vi "BonOMM-SAOMM.Test.vi"() -> ()   [LabVIEW 2011] (continued)
  in  "Port Local":u16
  in  "MCB Baud Rate":u32=57600
  out "Warning Code":u32
  in  "ANSW":string
  out "ActiveCmd":T15 caption="Commande Active"
  in  "TCS VRN":refnum<visa-resource-name>="COM7" caption="ID de connexion WinTCS"
  in  "PrAMS VRN":refnum<visa-resource-name>="COM4" caption="ID de connexion PrAMS"
  in  "MC-BonOMM VRN":refnum<visa-resource-name>="COM3"
  out "MCB COMM":bool=TRUE
  out "TCS COMM":bool=TRUE
  out "CmdPending":bool caption="Commande Active ?"
  out "CmdFIFO":T14(array[cluster]) caption="Commandes Latentes"
  out "Error Code":u32
  out "path_exclusion":path=path "C:/BonOMM/BonOMM 7.1/systemlogfiles" caption="Chemin du fichier d'exclusion"
  out "VI principal":path=path "C:/BonOMM/BonOMM 7.1/BonOMM 7.1.vi" caption="Chemin du dossier principal"
  out "path_config":path=path "C:/BonOMM/BonOMM 7.1/BonOMM 7.1.vi" caption="Répertoire de configuration"
  out "properties.ini":path=path "C:/BonOMM/BonOMM 7.1/BonOMM 7.1.vi" caption="Fichier de Configuration Système"
  out "instruments.ini":path=path "C:/BonOMM/BonOMM 7.1/BonOMM 7.1.vi" caption="Paramètres Instrumentaux"
  out "path_data":path=path "C:/BonOMM/BonOMM 7.1/systemlogfiles" caption="Répertoire de données"
  out "path_dss":path=path "C:/BonOMM/BonOMM 7.1/systemlogfiles" caption="Répertoire des données DSS"
  out "path_libdir":path=path "C:/BonOMM/BonOMM 7.1/systemlogfiles" caption="Répertoire des librairies d'objets"
  out "loaded_lib":path=path "C:/BonOMM/BonOMM 7.1/systemlogfiles" caption="Chemin vers la librairie chargée"
  out "path_SubVIs":path=path "C:/BonOMM/BonOMM 7.1/systemlogfiles" caption="Répertoire principal des sous routines"
  out "path_syslogs":path=path "C:/BonOMM/BonOMM 7.1/systemlogfiles" caption="Répertoire d'archivages principal"
  out "path_focuslog":path=path "C:/BonOMM/BonOMM 7.1/systemlogfiles" caption="Répertoire d'archivages des foyers instrumentaux"
  out "path_pointing":path=path "C:/BonOMM/BonOMM 7.1/systemlogfiles" caption="Répertoire d'archivages des pointés"
  out "path_trackfile":path=path "C:/BonOMM/BonOMM 7.1/tracklogfiles" caption="Répertoire d'archivage du guidage"
  out "path_Apps":path=path "C:/BonOMM/BonOMM 7.1/systemlogfiles" caption="Répertoire principal des applications externes"
  out "wgetexec":path=path "C:/BonOMM/BonOMM 7.1/systemlogfiles" caption="Chemin vers l'application wget.exe"
  out "IDLexec":path=path "C:/BonOMM/BonOMM 7.1/systemlogfiles" caption="Chemin vers l'application IDL"
  out "PrAMS COMM":bool=TRUE
  in  "Address du serveur":string
  out "Clients":string[](array[string]) caption="Clients TCP/IP"
  out "Clients ID":refnum<k5>[](array[refnum])
  in  "Hexapod VRN":refnum<visa-resource-name>="COM4" caption="ID de la connexion Hexapod Console"
  out "Calib COMM":bool=TRUE
  out "Calib VRN":refnum<visa-resource-name>="COM5" caption="Visa Ressource Name des lampes"
  in  "Calib Baud rate":u32=9600
  out "ExCmd COMM":bool=TRUE
  in  "Excmd VRN":refnum<visa-resource-name>="COM8"
  in  "Excmd Baud rate":u32=38400
  in  "Table Baud rate":u32=38400 caption="Baud Rate des tables"
  out "Table VRN":refnum<visa-resource-name>="COM9" caption="Visa Ressource Name des tables"
  out "TableCOM":bool=TRUE caption="Tables COMM"
  # "Paramètres"
  # "Control Emulation"
  # "Debug"
  # "Région d'intérêt"
  # "Tables de guidage"
  # "Foyers Télescope/Tables"
  # "Communications"
  # "Guidage"
  # "Falcon Processed"
  # "Position Hexapode"
  # "Position Nominale"
  # "Historique"
  # "X"
  # "Y"
  # "Z"
  # "U"
  # "V"
  # "Commandes"
  # "Offsets"
  # "Gains"
  # "Enabling Tab"
  # "Flags d'états"
  # "Variable d'applications"
  # "Propriétés de la fenêtre"
  # "Logs & Archives"
  # "Utilité à confirmer ..."
  # "Gestion des menus et librairies"
  # "Sauvegarde des Ctrls&Indics"
  # "Lampes de Calibration"
  # "Roues à Filtres"
  # "Caméra d'acquisition"
  # "Station Météo"
  # "Athermalisation des Foyers"
  # "LVDTs"
  # "À passer en commande de menu ..."
  # "Centre du Champ"
  # "TCS Status Bytes"
  # "Data USNO"
  # "À passer en commandes\ndu menu ..."
  # "Télescope (TCS & StarryNight)"
  # "Image de fond"
  # "Coordonnées Relatives"
  # "Centre du champ"
  # "Données USNO"
  # "Image DSS"
  # "Best Target"
  # "Bundles d'erreur"
  # "Temps d'exécution"
  # "Foyer"
  # "Prêt à pointer"
  # "En déplacement"
  # "Temps Univ."
  # "Entrainement"
  # "Temps Sidé."
  # "Angle Hor."
  # "Asc. Droite"
  # "Déclinaison"
  # "Époque"
  # "Air Mass"
  # "Télescope"
  # "Cible"
  # "Référence"
  # "OFFSET"
  # "Curseur"
  # "Z"
  # "Foyer (z)"
  # "X"
  # "Y"
  # "Z"
  # "U"
  # "V"
  # "Position"
  # "Écart"
  # "RA"
  # "DEC"
  # "Total"
  # "Sonde"
  # "Cible"
  # "Exposition"
  # "X"
  # "Y"
  # "Centroïds"
  # "Pixels"
  # "Résidu"
  # "''"
  # "Tmp(°)"
  # "Hum(%)"
  # "Ext."
  # "Int."
  # "Mir."
  # "Str."
  # "RA"
  # "DEC"
  # "Communications"
  # "Commandes Externes"
  # "Chemins système"
  # "Clients TCP/IP"
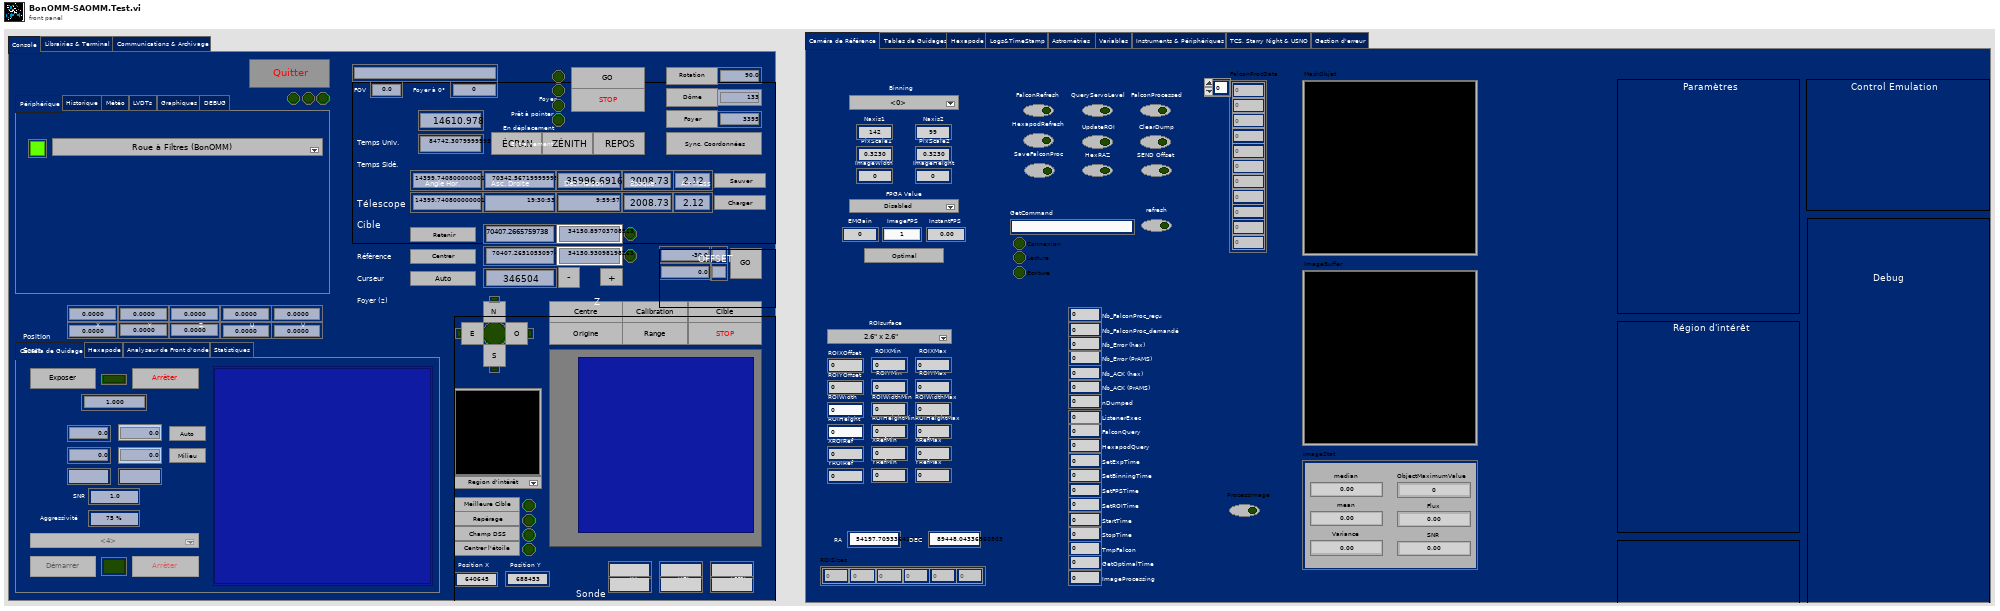
[diagram p1: front panel]
types:
  T1 = enum32{"Caméra de Référence", "Tables de Guidages", "Hexapode", "Logs&TimeStamp", "Astrométries", "Variables", "Instruments & Périphériques", "TCS, Starry Night & USNO", "Gestion d'erreur"}
  T2 = cluster{"median":dbl, "mean":dbl, "Variance":dbl, "ObjectMaximumValue":dbl, "Flux":dbl, "SNR":dbl}
  T3 = cluster{"Command Error":bool, "Slip/Stall":bool, "Overtravel":bool, "Done":bool, "nError":u32, "nSlip":u32, "nOT":u32, "nDone":u32}
  T4 = cluster{"NAXIS":dbl[], "CD":dbl[][], "CDELT":dbl[], "CRPIX":dbl[], "CTYPE":string[], "CRVAL":dbl[], "LONGPOLE":dbl, "LATPOLE":dbl, "PV2":dbl[]}
  T5 = typedef "LVPointTypeDef.ctl" = cluster{"Horizontal":i16, "Vertical":i16}
  T6 = typedef "LVRectTypeDef.ctl" = cluster{"Left":i16, "Top":i16, "Right":i16, "Bottom":i16}
  T7 = cluster{"Source":string, "Error Code":u32, "Warning Code":u32, "Comment":string}[]
  T8 = enum32{"Console", "Librairies & Terminal", "Communications & Archivage"}
  T9 = enum32{"Caméra de Guidage", "Hexapode", "Analyseur de Front d'onde", "Statistiques"}
  T10 = cluster{"X Values":dbl[], "Histogram: h(x)":i32[]}[]
  T11 = enum32{"Périphérique", "Historique", "Météo", "LVDTs", "Graphiques", "DEBUG"}
  T12 = cluster{"filtre #1":bool, "filtre #2":bool, "filtre #3":bool, "filtre #4":bool, "filtre #5":bool, "filtre #6":bool}
  T13 = cluster{"[Temp 1]":dbl, "[Temp 2]":dbl, "[Temp 3]":dbl, "[Temp 4]":dbl, "[Temp 5]":dbl, "[Temp 6]":dbl, "[Temp 7]":dbl, "[Temp 8]":dbl}
  T14 = cluster{"CmdAct":string, "CmdArgs":string, "Source":string}[]
  T15 = cluster{"CmdAct":string, "CmdArgs":string, "Source":string}
  T16 = enum32{"Console", "Librairies & Terminal", "Communications & Archivage", "Secondaire Actif"}
  T17 = enum8{"Enabled", "Disabled", "Disabled and Grayed Out"}
  T18 = cluster{"Source":string, "Error Code":i32, "Warning Code":i32, "Comment":string}[]
  T19 = cluster{"Command Error":bool, "Slip/Stall":bool, "Overtravel":bool, "Done":bool, "nError":dbl, "nSlip":dbl, "nOT":dbl, "nDone":dbl}
  T20 = cluster{"Invert Angle":bool, "Invert X":bool, "Invert Y":bool}
  T21 = cluster{"North Task":refnum<k21>, "West Task":refnum<k21>, "South Task":refnum<k21>, "East Task":refnum<k21>}
  T22 = cluster{"newFoyer":dbl, "updSonde":bool, "oldFoyer":dbl}
  T23 = cluster{"cRIO address":string, "Port Number":u16, "cRIO_commID":refnum<k5>, "Cx":bool}
  T24 = typedef "NI_LVConfig.lvlib/Config Data RefNum.ctl" = refnum<k1>
  T25 = cluster{"left":i16, "top":i16, "right":i16, "bottom":i16}
  T26 = typedef "LVRangeTypeDef.ctl" = cluster{"Minimum":dbl, "Maximum":dbl, "Increment":dbl, "Minor Increment":dbl, "Start":dbl}
  T27 = cluster{"PrAMS VRN":refnum<visa-resource-name>, "Signature":u32, "MessageType":cluster{string[], u32[]}, "Hexapod VRN":refnum<visa-resource-name>}
  T28 = cluster{"HexX":refnum<vi>, "HexY":refnum<vi>, "HexZ":refnum<vi>, "HexU":refnum<vi>, "HexV":refnum<vi>}
  T29 = cluster{"Angle Hor.":refnum<vi>, "DEC Tel":refnum<vi>, "Epoch Tel":refnum<vi>}
  T30 = cluster{"PrAMS actif":refnum<vi>, "PrAMS-ACK":refnum<vi>, "HexaCons actif":refnum<vi>, "Hexapod-ACK":refnum<vi>}
  T31 = cluster{"Offset X":refnum<vi>, "Offset Y":refnum<vi>, "Offset Z":refnum<vi>, "Offset U":refnum<vi>, "Offset V":refnum<vi>}
  T32 = cluster{"Calibration X":dbl, "Calibration Y":dbl}
  T33 = cluster{"Rangement X":dbl, "Rangement Y":dbl, "Rangement Z":dbl}
  T34 = cluster{"Calibration Y":dbl, "Calibration X":dbl}
  T35 = cluster{"Range Y":dbl, "Range X":dbl, "Range Z":dbl}
  T36 = cluster{"Cible X":refnum<vi>, "Cible Y":refnum<vi>, "Cible Z":refnum<vi>}
  T37 = cluster{"Table VRN":refnum<vi>, "Table Error":refnum<vi>, "Table actif":refnum<vi>}
  T38 = typedef "LVMouseTypeDef.ctl" = cluster{"Mouse Position":cluster{"X":i32, "Y":i32}, "Mouse Modifiers":cluster{"Button Down":bool, "Shift Mod":bool, "Menu Mod":bool, "Option Mod":bool}}
  T39 = typedef "LVBoundsTypeDef.ctl" = cluster{"Width":u32, "Height":u32}
  T40 = cluster{"TableAstrom":cluster{"NAXIS":dbl[], "CD":dbl[][], "CDELT":dbl[], "CRPIX":dbl[], "CTYPE":string[], "CRVAL":dbl[], "LONGPOLE":dbl, "LATPOLE":dbl, "PV2":dbl[]}, "FieldAstrom":cluster{"NAXIS":dbl[], "CD":dbl[][], "CDELT":dbl[], "CRPIX":dbl[], "CTYPE":string[], "CRVAL":dbl[], "LONGPOLE":dbl, "LATPOLE":dbl, "PV2":dbl[]}, "GuiderAstrom":cluster{"NAXIS":dbl[], "CD":dbl[][], "CDELT":dbl[], "CRPIX":dbl[], "CTYPE":string[], "CRVAL":dbl[], "LONGPOLE":dbl, "LATPOLE":dbl, "PV2":dbl[]}}
  T41 = cluster{"TCS VRN":refnum<visa-resource-name>, "TCS Error":errorcluster, "Table VRN":refnum<visa-resource-name>, "Table Error":errorcluster}
  T42 = cluster{"TCS actif":refnum<vi>, "Table actif":refnum<vi>, "Position Z":refnum<vi>, "StartServo":refnum<vi>, "Mode":refnum<vi>, "Servo":refnum<vi>, "StopServo":refnum<vi>, "DiffX":refnum<vi>, "DiffY":refnum<vi>, "SNR":refnum<vi>, "MovingXY":refnum<vi>}
  T43 = typedef "LVRowAndColumnTypeDef.ctl" = cluster{"Row":i32, "Column":i32}
  T44 = typedef "LVPointDoubleTypeDef.ctl" = cluster{"Cursor X":dbl, "Cursor Y":dbl}
  T45 = cluster{"name":string, "type desc":i16[], "flat data":string}[]
  T46 = typedef "gfitsio.lvlib/gfitsio-refnum.ctl" = refnum<k1>
  T47 = cluster{"Miroir":dbl, "Cursor.Cursor X":dbl, "Cursor.Cursor Y":dbl, "MirVig":dbl}
  T48 = typedef "LVPoint32TypeDef.ctl" = cluster{"Horizontal":i32, "Vertical":i32}
  T49 = cluster{"ROIXOffset OUT":u16, "ROIYOffset OUT":u16, "ROIWidth OUT":u16, "ROIHeight OUT":u16}
  T50 = cluster{"ROIXMin":u16, "ROIYXMax":u16, "ROIYMin":u16, "ROIYMax":u16}
  T51 = cluster{"ROIXOffset":u16, "ROIYOffset":u16, "ROIWidth":u16, "ROIHeight":u16}
  T52 = cluster{"Largeur de l'image":dbl, "Hauteur de l'image":dbl, "Bits par Pixel":dbl, "ID de l'image":u32, "Frame Rate":dbl, "Largeur de Bande":dbl, "Time Stamp":u64}
  T53 = cluster{"Largeur de la ROI":u16, "Hauteur de la ROI":u16, "Position X de la ROI":u16, "Position Y de la ROI":u16, "Minimum de la ROI":u32, "Maximum de la ROI":u32}
  T54 = cluster{"Seuil du masque":dbl, "Flux":dbl, "SNR":dbl, "Centroide X":dbl, "Centroide Y":dbl}
  T55 = cluster{"Logging ID":u32, "Logging TimeStapmp":u64, "Azimuth":dbl, "Elevation":dbl, "Rotation":dbl, "ServoLevel":u16, "ROIWidth":u16, "ROIHeight":u16, "ROIXOffset":u16, "ROIYOffset":u16, "Pixel X":dbl, "Pixel Y":dbl, "ImageTimeStamp":u64, "CommandTimeStamp":u64, "Flux":dbl, "SNR":dbl, "SNRTreshold":dbl, "CentroidX":dbl, "CentroidY":dbl}
  T56 = cluster{"Hexapod_Nominal":dbl[], "Hexapod_Offset":dbl[], "Hexapod_LUT":dbl[], "Hexapod_ServoX":dbl[], "Hexapode_ServoY":dbl[], "Hexapod_Console":dbl[], "Hexapod_Position":dbl[], "Hexapod_Command":dbl[], "Hexapod_Filtered":dbl[]}
  T57 = cluster{"SNR":dbl, "SNRTreshold":dbl, "Flux":dbl}
  T58 = cluster{"ServoLevel":u16, "ROIXOffset":u16, "CentroidX":dbl, "Pixel X":dbl, "ROIYOffset":u16, "CentroidY":dbl, "Pixel Y":dbl}
  T59 = enum16{"Left Button", "Center Button", "Right Button", "Window Close"}
  T60 = cluster{"GuidingCancel":refnum<vi>, "GuideNorth":refnum<vi>, "GuideSouth":refnum<vi>, "GuideEast":refnum<vi>, "GuideWest":refnum<vi>}
  T61 = cluster{"Commande":string, "Chaîne d'arguments":string, "Source":string}[]
  T62 = cluster{"Source":string, "Error Code":u32, "Warning Code":u32, "Comment":string}
  T63 = enum16{"fractional", "engineering", "exponential"}
  T64 = typedef "event.ctl" = cluster{"message":string, "data":variant}
diagram:
  # "Boucle principale: 8"
  # "Go on?"
  n1 = stacked-sequence {
    seq-local: [_ _ w80 _ _ _ _ _ _ _] -> [_ _ _ w203 w576 w714 w767 w800 w943 w7396]
    seq-local: [_ _ _ w201 _ _ _ _ _ _] -> [_ _ _ _ _ _ _ _ _ w7394]
    frame #0 {
      # "Lecture des fichiers \"controls.data\" et \"indicators.data\"\npour initialiser la face avant à son état sauvegarder ..."
      n2 = case shown="True" TRUE {
        frame True {
          # "Lecture du fichier de configuration dans lequel\nles variables sont toutes enregistrer quand on\nquitte le programme"
          n3 = Current VI's Path() -> (path=w3:path)
          n4 = Strip Path(path=w3) -> (stripped path=w4:path)  [unwired: 1 out]
          n5 = call <vilib>:"Get File Extension.vi"("file"=w4) -> ("lowercase file extension"=w5:string)  [unwired: 7 in, 3 out]
          n6 = case shown="\"exe\"" w5 {
            tunnel: w4 -> [w19 w21]
            tunnel: [w19 w20] -> w2
            frame Default {
            }
            frame "exe" {
              n7 = Strip Path(path=w21) -> (stripped path=w20:path)  [unwired: 1 out]
            }
          }
          n8 = global write "Globals.vi" "MasterDIR"(w2) -> ()
          n9 = Build Path(base path=w2, name or relative path="config") -> (appended path=w6:path)
          n10 = List Folder(path=w6) -> (filenames=w18:string[])  [unwired: 3 in, 3 out]
          n11 = Search 1D Array(1D array=w18, element="controls.data" ("name or relative path")) -> (index of element=w17:i32)  [unwired: 1 in]
          n12 = Search 1D Array(1D array=w18, element="indicators.data" ("name or relative path")) -> (index of element=w16:i32)  [unwired: 1 in]
          n13 = Greater Or Equal To 0?(x=w17) -> (x >= 0?=w15:bool)
          n14 = Greater Or Equal To 0?(x=w16) -> (x >= 0?=w14:bool)
          n15 = And(x=w15, y=w14) -> (x .and. y?=w13:bool)
          n16 = case shown="True" w13 {
            tunnel: w6 -> [_ w25]
            frame False {
              n17 = One Button Dialog(message="Impossible de trouver les fichiers d'initialisation ...") -> ()  [unwired: 1 in, 1 out]
            }
            frame True {
              n18 = Current VI's Path() -> (path=w26:path)
              n19 = Open VI Reference(vi path=w26) -> (vi reference=w32:refnum<vi>, error out=w31:errorcluster)  [unwired: 5 in]
              n20 = global write "Globals.vi" "BonOMM VI Refnum"(w32) -> ()
              n21 = flat-sequence {
                tunnel: [w45] -> w35
                tunnel: w32 -> [w44]
                tunnel: w31 -> [w43]
                tunnel: w27 -> [w36]
                tunnel: w35 -> [w68]
                tunnel: w23 -> [w59]
                frame #0 {
                  n22 = invoke class="VI" method="Ctrl Val.Get All"(reference=w44, error in=w43, "Controls"=TRUE ("controls")) -> (reference out=w46:refnum<vi>, error out=w37:errorcluster, "Get All Control Values Variant"=w48:cluster{"Name":string, "Variant Data":variant}[])  [unwired: 1 in, 1 out]
                  n23 = Unflatten From String(type=w48, binary string=w36) -> (value=w47:cluster{"Name":string, "Variant Data":variant}[])  [unwired: 3 in, 2 out]
                  n24 = for {
                    tunnel: w47 -> [w54] mode=indexing
                    tunnel: w46 -> [w58]
                    tunnel: w37 -> [w57]
                    tunnel: [w56] -> w45
                    tunnel: [w55] -> w41 mode=indexing
                    tunnel: [w53] -> w42 mode=indexing
                    n25 = Unbundle By Name(w54) -> ("Name"=w53:string, "Variant Data"=w52:variant)
                    n26 = invoke class="VI" method="Ctrl Val.Set"(reference=w58, error in=w57, "Control Name"=w53, "Value"=w52) -> (reference out=w56:refnum<vi>, error out=w55:errorcluster)  [unwired: 1 in, 3 out]
                  }
                  "CtrlName" <- w42
                  "CtrlSetError" <- w41
                  n27 = for {
                    tunnel: w41 -> [w51] mode=indexing
                    tunnel: [w50] -> w40 mode=indexing
                    n28 = Unbundle(w51) -> ("status"=w50:bool)  [unwired: 2 out]
                  }
                  n29 = Boolean Array To Number(Boolean array=w40) -> (number=w39:u32)
                  n30 = Greater Than 0?(x=w39) -> (x > 0?=→"CtrlGetErrInd":bool)
                }
                frame #1 {
                  n31 = invoke class="VI" method="Ctrl Val.Get All"(reference=w68, "Controls"=FALSE ("controls")) -> (reference out=w66:refnum<vi>, error out=w65:errorcluster, "Get All Control Values Variant"=w60:cluster{"Name":string, "Variant Data":variant}[])  [unwired: 2 in, 1 out]
                  n32 = Unflatten From String(type=w60, binary string=w59) -> (value=w67:cluster{"Name":string, "Variant Data":variant}[])  [unwired: 3 in, 2 out]
                  n33 = for {
                    tunnel: w67 -> [w74] mode=indexing
                    tunnel: w66 -> [w77]
                    tunnel: w65 -> [w76]
                    tunnel: [w75] -> w61 mode=indexing
                    n34 = Unbundle By Name(w74) -> ("Name"=w73:string, "Variant Data"=w72:variant)
                    n35 = invoke class="VI" method="Ctrl Val.Set"(reference=w77, error in=w76, "Control Name"=w73, "Value"=w72) -> (error out=w75:errorcluster)  [unwired: 1 in, 4 out]
                  }
                  "IndicSetError" <- w61
                  n36 = for {
                    tunnel: w61 -> [w71] mode=indexing
                    tunnel: [w70] -> w63 mode=indexing
                    n37 = Unbundle(w71) -> ("status"=w70:bool)  [unwired: 2 out]
                  }
                  n38 = Boolean Array To Number(Boolean array=w63) -> (number=w64:u32)
                  n39 = Greater Than 0?(x=w64) -> (x > 0?=→"IndicSetErrInd":bool)
                }
              }
              n40 = Build Path(base path=w25, name or relative path="indicators.data") -> (appended path=w24:path)
              n41 = Build Path(base path=w25, name or relative path="controls.data") -> (appended path=w28:path)
              n42 = call <vilib>:"Read Characters From File.vi"("file path (dialog if empty)"=w28, "convert eol? (no:F)"=FALSE) -> ("character string"=w27:string)  [unwired: 4 in, 3 out]
              n43 = call <vilib>:"Read Characters From File.vi"("file path (dialog if empty)"=w24, "convert eol? (no:F)"=FALSE) -> ("character string"=w23:string)  [unwired: 4 in, 3 out]
            }
          }
          n44 = control-ref of="TERMINAL"() -> (w8:refnum<vi>)
          n45 = control-ref of="Indicateur d'état"() -> (w9:refnum<vi>)
          n46 = call "TERMINAL.vi"("Indicateur Refnum"=w9, "Terminal Refnum"=w8, "Indicateur d'état"="Chargement des variables") -> ()
        }
        frame False {
        }
      }
    }
    frame #1 {
      w78 = FALSE
      n47 = local write "Quit"(w78) -> ()
      n48 = local write "Vérification des erreurs"(w78) -> ()
      n49 = local write "Lecture Configuration"(w78) -> ()
      n50 = local write "Gestion des menus"(w78) -> ()
      n51 = local write "Initialisation TCS"(w78) -> ()
      n52 = local write "Choix de l'insturment"(w78) -> ()
      n53 = local write "Vitesse des tables"(w78) -> ()
      n54 = local write "Astrométries"(w78) -> ()
      n55 = local write "PrAMS + Hexapode"(w78) -> ()
      n56 = local write "Connexion Météo"(w78) -> ()
      n57 = local write "Connexion LVDTs"(w78) -> ()
    }
    frame #2 {
      # "Ici sont listés les exceptions du chargement des variables\nLe tableau ci-dessous représente les variables dont la remise\nà l'état sauvegardée ne sera pas effectuée ... pour le modifier\nAllez dans l'onglet périphérique et cliquez sur \"Ajouter une exception de\nSauvegarde\""
      # "Lancement de CheckForError avant de faire quoique ce soit d'autre ..."
      n58 = local write "Indicateur d'état"("") -> ()
      n59 = local write "CameraSelector"(T9."Caméra de Guidage" ("CameraSelector")) -> ()
      n60 = local write "MainTab"(T16."Console" ("tab panel")) -> ()
      n61 = Current VI's Path() -> (path=w82:path)
      "VI principal" <- w82
      n62 = call "CheckForError.vi"("Main Path"=w82) -> ("Array of Folders"=w90:path[], "Array of Files"=w91:path[], "SkipInstr"=→"SkipChoixInstr":bool, "Bundle-Meteo"=w92:T23, "This VI's Path"=w85:path, "term"=w87:string, "Go on ?"=w80:bool, "Array of Baud Rates"=w93:u32[], "Array of VISA refnum"=w94:refnum<visa-resource-name>[], "Serial"=w86:bool[])  [unwired: 3 in, 2 out]
      n63 = case shown="True" w80 {
        tunnel: w94 -> [_ w155]
        tunnel: w93 -> [_ w154]
        tunnel: w92 -> [_ w153]
        tunnel: w91 -> [_ w152]
        tunnel: w90 -> [_ w151]
        tunnel: w87 -> [_ w139]
        tunnel: w86 -> [_ w136]
        tunnel: w85 -> [_ w125]
        frame False {
        }
        frame True {
          # "En changeant ça pour un bundle nommé, on éviterait bien des problèmes ..."
          # "En attendant on utilise les valeurs suivantes ..."
          n64 = Index Array(array=w151) -> (element #1=→"path_config":path, element #2=→"path_data":path, element #3=→"path_libdir":path, element #4=→"path_dss":path, element #5=w96:path, element #6=→"path_syslogs":path, element #7=→"path_focuslog":path, element #8=→"path_pointing":path, element #9=→"path_trackfile":path, element #10=→"path_Apps":path)  [unwired: 10 in]
          "path_SubVIs" <- w96
          n65 = Index Array(array=w152) -> (element #1=→"properties.ini":path, element #2=→"instruments.ini":path, element #5=→"loaded_lib":path, element #6=→"IDLexec":path, element #7=→"wgetexec":path)  [unwired: 7 in, 2 out]
          n66 = Unbundle By Name(w153) -> ("cRIO address"=w122:string, "Port Number"=w121:u16, "cRIO_commID"=→"cRIO_commID":refnum<k5>, "Cx"=w123:bool)
          "cRIO address" <- w122
          "cRIO Port" <- w121
          "Cx" <- w123
          n67 = Open VI Reference(vi path=w125) -> (vi reference=w124:refnum<vi>, error out=w115:errorcluster)  [unwired: 5 in]
          n68 = Index Array(array=w155) -> (element #1=w158:refnum<visa-resource-name>, element #2=w111:refnum<visa-resource-name>, element #3=w110:refnum<visa-resource-name>, element #4=w109:refnum<visa-resource-name>, element #5=w102:refnum<visa-resource-name>, element #6=w104:refnum<visa-resource-name>, element #7=w103:refnum<visa-resource-name>, element #8=w101:refnum<visa-resource-name>)  [unwired: 8 in]
          n69 = Index Array(array=w136) -> (element #1=→"TableCOM":bool, element #2=→"PrAMS COMM":bool, element #3=→"TCS COMM":bool, element #4=→"Calib COMM":bool, element #5=→"ExCmd COMM":bool, element #6=→"MCB COMM":bool)  [unwired: 6 in]
          n70 = Index Array(array=w154) -> (element #1=w157:u32, element #2=w108:u32, element #3=w107:u32, element #4=w106:u32)  [unwired: 5 in, 1 out]
          n71 = property class="VI"(reference=w124, error in=w115) -> (reference out=w116:refnum<vi>, error out=w114:errorcluster, "Front Panel.Open"=w113:bool)
          n72 = local write "MC-BonOMM VRN"(w109) -> ()
          n73 = local write "PrAMS VRN"(w103) -> ()
          n74 = local write "Table VRN"(w158) -> ()
          n75 = local write "Calib VRN"(w111) -> ()
          n76 = local write "Excmd VRN"(w110) -> ()
          n77 = local write "Splitter VRN"(w102) -> ()
          n78 = local write "Hexapod VRN"(w101) -> ()
          n79 = local write "TCS VRN"(w104) -> ()
          n80 = case shown="True" w113 {
            tunnel: w116 -> [_ w188]
            tunnel: w114 -> [w185 w187]
            tunnel: [w185 w186] -> w112
            frame False {
            }
            frame True {
              n81 = invoke class="VI" method="FP.Close"(reference=w188, error in=w187) -> (error out=w186:errorcluster)  [unwired: 1 in, 2 out]
            }
          }
          n82 = local write "Excmd Baud rate"(w107) -> ()
          n83 = local write "Table Baud rate"(w157) -> ()
          n84 = local write "Calib Baud rate"(w108) -> ()
          n85 = local write "MCB Baud Rate"(w106) -> ()
          n86 = String To IP() -> (0:w129:u32)  [unwired: 1 in]
          n87 = local write "VI Reference Error"(w112) -> ()
          n88 = IP To String(1:TRUE ("dot notation? (F)"), 2:w129) -> (0:w128:string)
          n89 = control-ref of="TERMINAL"() -> (w160:refnum<vi>)
          n90 = control-ref of="Indicateur d'état"() -> (w159:refnum<vi>)
          n91 = local write "Address du serveur"(w128) -> ()
          n92 = local write "Port Local"(u16 8380 ("Port Local")) -> ()
          n93 = call "TERMINAL.vi"("Indicateur Refnum"=w159, "Terminal Refnum"=w160, "Indicateur d'état"=w139) -> ()
          n94 = disable-structure shown="Enabled" {
            disable-tunnel: [w183 string[][] [] ("Output Table")] -> w120
            disable-tunnel: path "" ("Path") -> [w182 _]
            frame Disabled {
              n95 = call "Read_obs_files.vi"("Path"=w182) -> ("Output Table"=w183:string[][])  [unwired: 1 out]
            }
            frame Enabled {
            }
          }
          n96 = local read "LST"() -> (w119:dbl)
          n97 = Build Path(base path=w96, name or relative path="GUI\\InitProgress.vi") -> (appended path=w97:path)
          n98 = disable-structure shown="Disabled" {
            disable-tunnel: w123 -> [w163 _]
            disable-tunnel: w122 -> [w162 _]
            disable-tunnel: w121 -> [w161 _]
            frame Disabled {
              n99 = case shown="True" w163 {
                tunnel: w162 -> [_ w167]
                tunnel: w161 -> [_ w166]
                frame False {
                }
                frame True {
                  w164 = FALSE
                  w165 = FALSE
                  n100 = case shown="True" w165 {
                    tunnel: w167 -> [_ w176]
                    tunnel: w166 -> [_ w175]
                    frame False {
                    }
                    frame True {
                      n101 = TCP Open Connection(address=w176, remote port or service name=w175) -> (connection ID=w174:refnum<k5>, error out=→"Meteo Error":errorcluster)  [unwired: 3 in]
                      n102 = local write "cRIO_commID"(w174) -> ()
                    }
                  }
                  n103 = case shown="True" w164 {
                    frame False {
                    }
                    frame True {
                      n104 = shared-variable-open(refnum<k21> "ni.var.psp://132.204.61.43/varlib/LVDT-RA" ("shared variable refnum in"), dbl[] [], 5000 ("timeout ms")) -> (→"LVDT-RA":refnum<k21>, w172:errorcluster)  [unwired: 3 in]
                      n105 = local write "LVDT Error"(w172) -> ()
                    }
                  }
                  "Connexion LVDTs" <- w164
                  "Connexion Météo" <- w165
                }
              }
            }
            frame Enabled {
            }
          }
          n106 = for {
            tunnel: w120 -> [w194] mode=indexing
            tunnel: w119 -> [w195]
            tunnel: [w191] -> w117 mode=indexing
            n107 = Index Array(array=w194, index #1=2 ("index"), index #2=3 ("index")) -> (element #1=w197:string, element #2=w196:string)
            n108 = call "Airmass.vi"("temps sidéral"=w195, "DEC"=w196, "RA"=w197) -> ("airmass"=w192:dbl)
            n109 = Number To Fractional String(number=w192, precision (6)=i16 2) -> (F-format string=w193:string)  [unwired: 2 in]
            n110 = Insert Into Array(array=w194, index=5, new element=w193) -> (w191:string[])
          }
          n111 = Open VI Reference(vi path=w97) -> (vi reference=w99:refnum<vi>)  [unwired: 5 in, 1 out]
          n112 = flat-sequence {
            tunnel: w99 -> [w178]
            tunnel: [w178] -> w100
            tunnel: w100 -> [w180]
            frame #0 {
              n113 = local write "QuitInitialization"(FALSE ("QuitInitialization")) -> ()
            }
            frame #1 {
              n114 = control-ref of="QuitInitialization"() -> (w179:refnum<vi>)
              n115 = call "InitProgressLauncher.vi"("InitProgRef"=w180, "EscapeRef"=w179) -> ()  [unwired: 14 in]
            }
            frame #2 {
              n116 = disable-structure shown="Disabled" {
                frame Disabled {
                  n117 = Wait (ms)(milliseconds to wait=u32 500) -> ()  [unwired: 1 out]
                }
                frame Enabled {
                }
              }
            }
          }
          n118 = local write "Librairie des objets"(w117) -> ()
          n119 = local write "Librairie complète"(w117) -> ()
          "Vérification des erreurs" <- FALSE ("Vérification des erreurs")
        }
      }
      "Exception" <- "Tableau des exceptions"
      "NeedOrigin" <- TRUE ("NeedOrigin")
    }
    frame #3 {
      w202 = FALSE
      w200 = TRUE ("Visible")
      w201 = FALSE ("ShowAllHidden")
      # "Si jamais il y en a plus, il faudra gérer leur emplacement de\nfaçon \"programmatique\""
      # "Les 6 alarmes principales"
      # "Anciennement cachés"
      # "Ici on initialise les boutons et variables qui sont constants\net ne dépendent de l'état enregistrer ..."
      # "Pour montrer tout les indicateurs et contrôles \nqui sont normalement caché, changé la constante \nà vrai et faîtes rouler le programme une fois."
      n120 = case shown="True" w203 {
        frame False {
        }
        frame True {
          w215 = FALSE ("Visible")
          w216 = FALSE
          w207 = "communications"
          w258 = "hexapode"
          w302 = "Gains" ("section")
          w249 = "guidage"
          w260 = "camera"
          w373 = u16 2 items=["Region d'intérêt", "Prévisualisation", "Idle"] ("ImageUsage")
          w406 = "LVDTs" ("key")
          w413 = ""
          w421 = T17."Enabled" ("Disabled")
          w444 = u16 4 items=["Roue à Filtres (BonOMM)", "Roue à Filtres (PANO-II)", "Foyer ST-133", "Lampes d'étalonnage", "Options des périphériques"] ("Périphérique")
          w234 = TRUE
          w454 = T17."Enabled" ("Disabled")
          w461 = errorcluster {"status"=FALSE, "code"=0, "source"=""} ("Serial Error")
          w473 = FALSE
          w382 = "tables"
          w222 = "variables"
          w516 = 0
          w518 = 0.0
          w519 = 0.0
          w425 = -inf
          w525 = T17."Disabled" ("Disabled")
          w531 = u8 2 ("X Scale.Scale Fit")
          w532 = FALSE
          w529 = FALSE
          w397 = TRUE
          w233 = FALSE
          # "Initialisation de l'état des contrôles des roues à filtres"
          # "Initialise les boutons booléens à Faux"
          n121 = local read "properties.ini"() -> (w511:path)
          n122 = local write "Événements Software"(w233) -> ()
          n123 = local write "Synchro StarryNight"(w233) -> ()
          n124 = local write "Événements Usagés"(w233) -> ()
          n125 = local write "Archivage SAOMM"(w233) -> ()
          n126 = local write "Afficahge d'erreur"(w233) -> ()
          n127 = local write "PrAMS + SAOMM"(w233) -> ()
          n128 = local write "Hexapod Listener"(w233) -> ()
          n129 = local write "Query et Status"(w233) -> ()
          n130 = local write "PrAMS Listener"(w233) -> ()
          n131 = local write "Scripts Listener"(w233) -> ()
          n132 = local write "Gestion Scripts"(w233) -> ()
          n133 = local write "Guidage"(w233) -> ()
          n134 = call <vilib>:"Open Config Data.vi"("create file if necessary (T)"=FALSE, "configuration file path"=w511) -> ("error out"=w474:errorcluster, "refnum"=w475:T24)  [unwired: 7 in, 1 out]
          n135 = local write "Stops"(w233) -> ()
          n136 = local write "ActiveStages"(string[] ["AX", "AY", "AZ"] ("ActiveStageTag")) -> ()
          n137 = call-poly <vilib>:"Read Key.vi"("section"=w222, "error in (no error)"=w474, "key"="k0_focus", "refnum"=w475) -> ("error out"=w483:errorcluster, "value"=w478:dbl, "refnum out"=w482:T24)  [unwired: 4 in, 1 out]
          n138 = local write "k0_focus"(w478) -> ()
          n139 = call-poly <vilib>:"Read Key.vi"("section"=w222, "error in (no error)"=w483, "key"="k1_focus", "refnum"=w482) -> ("error out"=w484:errorcluster, "value"=w477:dbl, "refnum out"=w485:T24)  [unwired: 4 in, 1 out]
          n140 = local write "StopCam"(w233) -> ()
          n141 = local write "GoCam"(w233) -> ()
          n142 = local write "k1_focus"(w477) -> ()
          n143 = local write "Range"(w233) -> ()
          n144 = local write "Offset OK"(w233) -> ()
          n145 = local write "ModCoor"(w233) -> ()
          n146 = local write "StopTel"(w233) -> ()
          n147 = local write "Synctel"(w233) -> ()
          n148 = local write "Zénith"(w233) -> ()
          n149 = local write "Écran"(w233) -> ()
          n150 = local write "GO"(w233) -> ()
          n151 = call-poly <vilib>:"Read Key.vi"("section"=w222, "error in (no error)"=w484, "key"="a1_focus", "refnum"=w485) -> ("error out"=w486:errorcluster, "value"=w481:dbl, "refnum out"=w487:T24)  [unwired: 4 in, 1 out]
          n152 = local write "a1_focus"(w481) -> ()
          n153 = local write "ModifDome"(w233) -> ()
          n154 = local write "ModifRotation"(w233) -> ()
          n155 = local write "Coupole-Tél"(w233) -> ()
          n156 = local write "ModifFoyer"(w233) -> ()
          n157 = local write "act_cible"(w216) -> ()
          n158 = local write "act_sonde"(w234) -> ()
          n159 = local write "FirstBest"(w234) -> ()
          n160 = local write "ApplyCorrection"(w233) -> ()
          n161 = local write "TableMute"(w216) -> ()
          n162 = call-poly <vilib>:"Read Key.vi"("section"=w222, "error in (no error)"=w486, "key"="a2_focus", "refnum"=w487) -> ("error out"=w489:errorcluster, "value"=w480:dbl, "refnum out"=w488:T24)  [unwired: 4 in, 1 out]
          n163 = local write "a2_focus"(w480) -> ()
          n164 = local write "TCSMute"(w216) -> ()
          n165 = call-poly <vilib>:"Read Key.vi"("section"=w222, "error in (no error)"=w489, "key"="a3_focus", "refnum"=w488) -> ("error out"=w239:errorcluster, "value"=w479:dbl, "refnum out"=w240:T24)  [unwired: 4 in, 1 out]
          n166 = local write "a3_focus"(w479) -> ()
          n167 = local write "BestCount"(0 ("BestCount")) -> ()
          n168 = local write "ReconnectionMute"(w216) -> ()
          n169 = property on="DS9" class="Bool (strict)"("DisabledEnum"=w421) -> ()  [unwired: 2 in, 2 out]
          n170 = property on="best_target" class="Bool (strict)"("DisabledEnum"=w421) -> ()  [unwired: 2 in, 2 out]
          n171 = call-poly <vilib>:"Read Key.vi"("section"=w222, "error in (no error)"=w239, "default value"=2000.0, "key"="equinox", "refnum"=w240) -> ("error out"=w227:errorcluster, "value"=→"dflt-EQX":dbl, "refnum out"=w228:T24)  [unwired: 3 in, 1 out]
          n172 = local write "Bypass Auto-focus"(w233) -> ()
          n173 = local write "PrAMS COMM"(w233) -> ()
          n174 = local write "ImageDSSLed"(w233) -> ()
          n175 = local write "CentrageLed"(w233) -> ()
          n176 = local write "BestTargetLed"(w233) -> ()
          n177 = local write "TCS COMM"(w233) -> ()
          n178 = local write "CursorLock"(w233) -> ()
          n179 = local write "USNO_ready"(w233) -> ()
          n180 = local write "LVDT-Save-Data"(w233) -> ()
          n181 = local write "DSS_ready"(w233) -> ()
          n182 = local write "DSS_ready"(w233) -> ()
          n183 = local write "DS9-Led"(w233) -> ()
          n184 = local write "Déplacement usager"(w233) -> ()
          n185 = local write "FIFO d'erreur"(T18 [] ("FIFO d'erreur")) -> ()
          n186 = local write "stoptable"(w233) -> ()
          n187 = local write "Quit"(w233) -> ()
          n188 = call-poly <vilib>:"Read Key.vi"("section"=w222, "error in (no error)"=w227, "key"="mirror", "refnum"=w228) -> ("error out"=w225:errorcluster, "value"=→"Miroir":dbl, "refnum out"=w226:T24)  [unwired: 4 in, 1 out]
          n189 = global write "Globals.vi" "EXIT"(w233) -> ()
          n190 = call-poly <vilib>:"Read Key.vi"("section"=w222, "error in (no error)"=w225, "key"="mirvig", "refnum"=w226) -> ("error out"=w218:errorcluster, "value"=→"MirVig":dbl, "refnum out"=w219:T24)  [unwired: 4 in, 1 out]
          n191 = control-ref of="TERMINAL"() -> (w528:refnum<vi>)
          n192 = control-ref of="Indicateur d'état"() -> (w527:refnum<vi>)
          n193 = local write "ApplyCorrection"(w233) -> ()
          n194 = local read "Offset DEC"() -> (w450:dbl)
          n195 = local read "Offset RA"() -> (w451:dbl)
          n196 = call-poly <vilib>:"Read Key.vi"("section"=w406, "error in (no error)"=w218, "key"="ra-zero", "refnum"=w219) -> ("error out"=w408:errorcluster, "value"=w402:dbl, "refnum out"=w410:T24)  [unwired: 4 in, 1 out]
          n197 = property on="OffDEC_dir" class="Str"("DisabledEnum"=w525) -> ()  [unwired: 2 in, 2 out]
          n198 = local write "LVDT-zero"(w402) -> ()
          n199 = local write "VarTab"(T1."Variables" ("VarTab")) -> ()
          n200 = property on="Obslib" class="Tbl (strict)"("Visible Items:Row Headers Visible"=w529, "Visible Items:Column Headers Visible"=w397, "Visible Items:Vertical Scrollbar Visible"=w529, "Visible Items:Horizontal Scrollbar Visible"=w529) -> ()  [unwired: 2 in, 2 out]
          n201 = property on="Librairie des objets" class="Tbl (strict)"("Visible Items:Row Headers Visible"=w529, "Visible Items:Column Headers Visible"=w397, "Visible Items:Vertical Scrollbar Visible"=w397, "Visible Items:Horizontal Scrollbar Visible"=w529) -> ()  [unwired: 2 in, 2 out]
          n202 = local write "Périphérique"(w444) -> ()
          n203 = call "TERMINAL.vi"("Indicateur Refnum"=w527, "Terminal Refnum"=w528, "Indicateur d'état"="Initialisation des variables") -> ()
          n204 = call "Set_Offset_dir.vi"("DEC"=w450, "RA"=w451) -> ("DEC_dir"=w453:string, "RA_dir"=w452:string)
          n205 = local write "Focusing"(w233) -> ()
          n206 = call-poly <vilib>:"Read Key.vi"("section"=w406, "error in (no error)"=w408, "key"="ra-scale", "refnum"=w410) -> ("error out"=w407:errorcluster, "value"=w401:dbl, "refnum out"=w409:T24)  [unwired: 4 in, 1 out]
          n207 = local write "LVDT-scale"(w401) -> ()
          n208 = property on="OffRA_dir" class="Str"("DisabledEnum"=w525) -> ()  [unwired: 2 in, 2 out]
          n209 = local write "OffDEC_dir"(w453) -> ()
          n210 = local write "OffRA_dir"(w452) -> ()
          n211 = call-poly <vilib>:"Read Key.vi"("section"=w406, "error in (no error)"=w407, "key"="acq-time", "refnum"=w409) -> ("error out"=w261:errorcluster, "value"=w400:dbl, "refnum out"=w259:T24)  [unwired: 4 in, 1 out]
          n212 = local write "LVDT-time"(w400) -> ()
          n213 = property on="ChoixFiltre" class="Clust (strict)"() -> ("Controls[]"=w545:refnum<vi>[])  [unwired: 2 in, 2 out]
          n214 = call-poly <vilib>:"Read Key.vi"("section"=w260, "error in (no error)"=w261, "default value"=1000, "key"="naxis1", "refnum"=w259) -> ("error out"=w371:errorcluster, "value"=w324:u32, "refnum out"=w369:T24)  [unwired: 3 in, 1 out]
          n215 = Index Array(array=w545, index #1=0 ("indice"), index #2=1 ("indice"), index #3=2 ("indice"), index #4=3 ("indice"), index #5=4 ("indice"), index #6=5 ("indice")) -> (element #1=w543:refnum<vi>, element #2=w542:refnum<vi>, element #3=w541:refnum<vi>, element #4=w540:refnum<vi>, element #5=w539:refnum<vi>, element #6=w538:refnum<vi>)
          n216 = call-poly <vilib>:"Read Key.vi"("section"=w260, "error in (no error)"=w371, "default value"=1000, "key"="naxis2", "refnum"=w369) -> ("error out"=w370:errorcluster, "value"=w325:u32, "refnum out"=w368:T24)  [unwired: 3 in, 1 out]
          n217 = property class="Ctl"(reference=w543, "Blinking"=w532) -> ()  [unwired: 1 in, 2 out]
          n218 = property class="Ctl"(reference=w542, "Blinking"=w532) -> ()  [unwired: 1 in, 2 out]
          n219 = property class="Ctl"(reference=w541, "Blinking"=w532) -> ()  [unwired: 1 in, 2 out]
          n220 = property class="Ctl"(reference=w540, "Blinking"=w532) -> ()  [unwired: 1 in, 2 out]
          n221 = property class="Ctl"(reference=w539, "Blinking"=w532) -> ()  [unwired: 1 in, 2 out]
          n222 = property class="Ctl"(reference=w538, "Blinking"=w532) -> ()  [unwired: 1 in, 2 out]
          n223 = call-poly <vilib>:"Read Key.vi"("section"=w260, "error in (no error)"=w370, "key"="pixscale1", "refnum"=w368) -> ("error out"=w372:errorcluster, "value"=w356:dbl, "refnum out"=w367:T24)  [unwired: 4 in, 1 out]
          n224 = property on="Écran" class="Bool (strict)"("DisabledEnum"=w454) -> ()  [unwired: 2 in, 2 out]
          n225 = property on="Zénith" class="Bool (strict)"("DisabledEnum"=w454) -> ()  [unwired: 2 in, 2 out]
          n226 = property on="Range" class="Bool (strict)"("DisabledEnum"=w454) -> ()  [unwired: 2 in, 2 out]
          n227 = property on="ModifRotation" class="Bool (strict)"("DisabledEnum"=w454) -> ()  [unwired: 2 in, 2 out]
          n228 = property on="ModifDome" class="Bool (strict)"("DisabledEnum"=w454) -> ()  [unwired: 2 in, 2 out]
          n229 = property on="ModifFoyer" class="Bool (strict)"("DisabledEnum"=w454) -> ()  [unwired: 2 in, 2 out]
          n230 = property on="Synctel" class="Bool (strict)"("DisabledEnum"=w454) -> ()  [unwired: 2 in, 2 out]
          n231 = property on="ModCoor" class="Bool (strict)"("DisabledEnum"=w454) -> ()  [unwired: 2 in, 2 out]
          n232 = property on="SaveCoords" class="Bool (strict)"("DisabledEnum"=w454) -> ()  [unwired: 2 in, 2 out]
          n233 = property on="GO" class="Bool (strict)"("DisabledEnum"=w454) -> ()  [unwired: 2 in, 2 out]
